vi "ProjectClose.vi"(8 "error in (no error)":errorcluster) -> (0 "error out":errorcluster)   [LabVIEW 2020, in "ni-veristand-steps-runtime-lib.lvlib"]
uses:
  ni-veristand-steps-runtime-lib.lvlib
  <vilib>/NI VeriStand/Execution/Project/NI_VS Project ExecutionAPI.lvlib
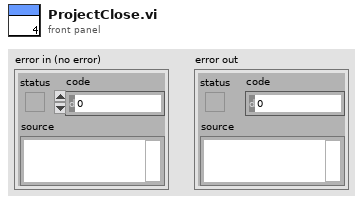
[diagram p1: front panel]
types:
  T1 = typedef "ni-veristand-steps-runtime-lib.lvlib/VeriStand dotNet References.ctl" = cluster{"ModelManager":T2, "AlarmManager":T3, "ChannelFault":T4, "WorkspaceManager":T5, "Project Ref":T6}
  T2 = typedef "NI_VS ModelManager ExecutionAPI.lvlib/ModelManagerAPI.ctl" = refnum<k24>
  T3 = typedef "NI_VS AlarmManager ExecutionAPI.lvlib/AlarmManagerAPI.ctl" = refnum<k24>
  T4 = typedef "NI_VS ChannelFault ExecutionAPI.lvlib/ChannelFaultAPI.ctl" = refnum<k24>
  T5 = typedef "NI_VS Workspace ExecutionAPI.lvlib/WorkspaceAPI.ctl" = refnum<k24>
  T6 = typedef "NI_VS Project ExecutionAPI.lvlib/Project Ref.ctl" = refnum<k24>
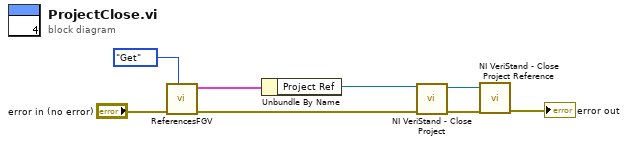
[diagram p0: block diagram]
diagram:
  n1 = call "ReferencesFGV.vi"("Get/Set"=enum16{"Get", "Set"}."Get", "error in (no error)"="error in (no error)") -> ("error out"=w5:errorcluster, "VeriStand dotNET Refs out"=w2:T1)  [unwired: 8 in]
  n2 = Unbundle By Name(w2) -> ("Project Ref"=w1:T6)
  n3 = call <vilib>:"NI VeriStand - Close Project.vi"("error in (no error)"=w5, "Project Ref in"=w1) -> ("error out"=w7:errorcluster, "Project Ref out"=w8:T6)  [unwired: 8 in]
  n4 = call <vilib>:"NI VeriStand - Close Project Reference.vi"("error in (no error)"=w7, "Project Ref"=w8) -> ("error out"=→"error out":errorcluster)  [unwired: 9 in]
